vi "Test Boolean Event.vi"() -> ()   [LabVIEW 2021]
uses:
  Source/Omni-Bus/Omni_Bus.lvclass
  Source/Event Bus/Event_Bus.lvclass
  C:/TSA/Omni-Bus/Source/Omni-Bus/Bus Access/Bus_Access.lvclass
  Source/Local Bus/Local Bus.lvclass
  Source/Local Bus/Support/Tag List Type.ctl
  <vilib>/Utility/Data Type/Type Definitions/Data Type.ctl
  <vilib>/TSA/Abstract Data Classes/Abs_Types/Type/Abs_Type.lvclass/Abs_Type.ctl
  Source/Omni-Bus/Omni_Bus.lvclass/Omni_Bus.ctl
  Source/Omni-Bus/Support/Write/Write Boolean.vi
  Source/Omni-Bus/Support/Read/Read Boolean.vi
  Source/Omni-Bus/Support/FindVar.vi
  <vilib>/Utility/error.llb/Clear Errors.vi
  Source/Omni-Bus/Properties/Read Var Map.vi
  <vilib>/TSA/Abstract Data Classes/Abs_Types/Type/Properties/Read Tag.vi
  <vilib>/TSA/Abstract Data Classes/Abs_Types/Boolean/Abs_Boolean.lvclass
  C:/Program Files (x86)/National Instruments/LabVIEW 2021/vi.lib/TSA/Abstract Data Classes/Abs_Types/Type/Abs_Type.lvclass
  <vilib>/TSA/Abstract Data Classes/Abs_Types/Value/Abs_Value.lvclass
  Source/Omni-Bus/Support/Check For Read Only Error.vi
  Source/Omni-Bus/Support/Incorrect Tag String Error.vi
  <vilib>/TSA/Abstract Data Classes/Abs_Types/Type/Abs_Type.lvclass
  <vilib>/Utility/Data Type/NI_Data Type.lvlib
panel:
  in  "stop 6":bool
  out "Numeric 6":i32
  in  "Boolean 6":bool
  in  "stop 5":bool
  out "Numeric 5":i32
  out "Boolean 5":bool
  in  "stop 4":bool
  out "Numeric 4":i32
  out "Boolean 4":bool
  in  "stop 3":bool
  out "Numeric 3":i32
  out "Boolean 3":bool
  out "Boolean 2":bool
  in  "Boolean":bool
  out "Numeric 2":i32
  out "Numeric":i32
  in  "stop 2":bool
  in  "stop":bool
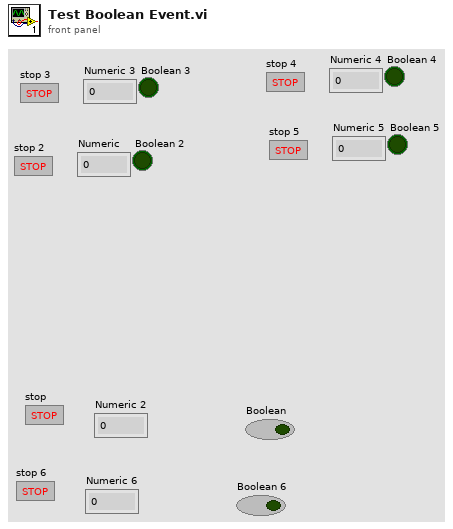
[diagram p1: front panel]
types:
  T1 = typedef "Local Bus.lvclass/Tag List Type.ctl" = cluster{"Tag":string, "Type":T2}
  T2 = typedef "NI_Data Type.lvlib/Data Type.ctl" = enum8{"Invalid Type", "Void", "I8", "I16", "I32", "I64", "U8", "U16", "U32", "U64", "Single Float", "Double Float", "Extended Float", "Single Complex", "Double Complex", "Extended Complex", "Enum U8", "Enum U16", "Enum U32", "Enum U64", "Single Float With Unit", "Double Float With Unit", "Extended Float With Unit", "Single Complex with Unit", "Double Complex with Unit", "Extended Complex with Unit", "Boolean", "String", "Path", "Picture", "Tag", "Array", "Cluster", "Variant", "LV Variant", "Waveform", "Timestamp", "Digital Waveform", "Digital Data", "ExpressData", "Refnum", "External Data", "VI", "Poly VI", "LabVIEW Class Instance", "Fixed Point", "Set Collection", "Map Collection"}
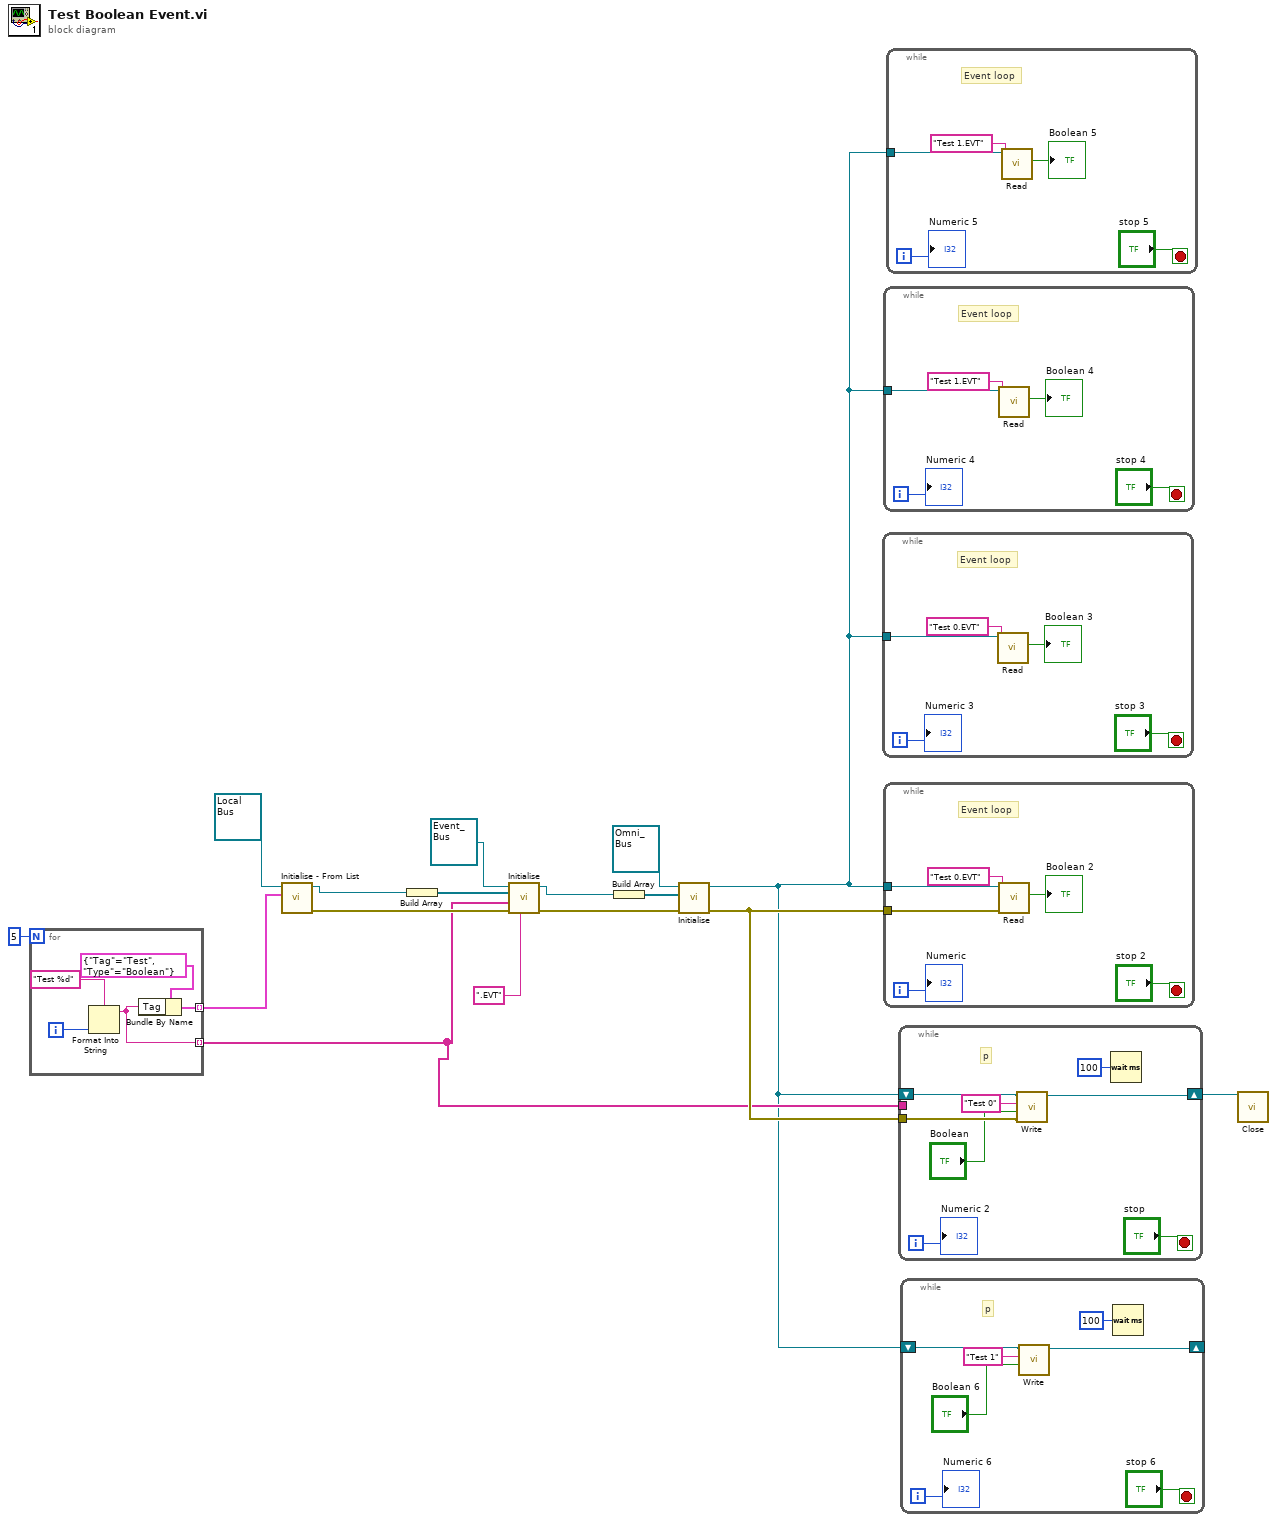
[diagram p0: block diagram]
diagram:
  n1 = for {
    N: 5 -> [_]
    tunnel: [w18] -> w4 mode=indexing
    tunnel: [w17] -> w3 mode=indexing
    i -> [w19]
    n2 = Format Into String(format string="Test %d", w19) -> (resulting string=w17:string)  [unwired: 2 in, 1 out]
    n3 = Bundle By Name(cluster=T1 {"Tag"="Test", "Type"=enum."Boolean"} ("Cluster"), "Tag"=w17) -> (w18:T1)
  }
  n4 = call "Initialise - From List.vi"("Tag List"=w4, "Local Bus in"=refnum<class "Local Bus.lvclass"> refnum) -> ("error out"=w9:errorcluster, "Local Bus out"=w8:refnum<class "Local Bus.lvclass">)  [unwired: 8 in]
  n5 = Build Array(w8) -> (w10:refnum<class "Local Bus.lvclass">[])
  n6 = call "Initialise.vi"("Tag Root"=".EVT", "error in (no error)"=w9, "Tags to Event"=w3, "Buses"=w10, "Event_Bus in"=refnum<class "Event_Bus.lvclass"> refnum) -> ("error out"=w13:errorcluster, "Event_Bus out"=w12:refnum<class "Event_Bus.lvclass">)  [unwired: 5 in]
  n7 = Build Array(w12) -> (w14:refnum<class "Event_Bus.lvclass">[])
  n8 = call-dynamic "Initialise.vi"("error in (no error)"=w13, "Bus Access"=w14, "Var Bus in"=refnum<class "Omni_Bus.lvclass"> refnum) -> ("error out"=w15:errorcluster, "Var Bus out"=w1:refnum<class "Omni_Bus.lvclass">)  [unwired: 7 in]
  n9 = while {
    tunnel: w1 -> [w26]
    i -> [w24]
    stop <- "stop 3" stop-if-true
    # "Event loop"
    n10 = call-poly "Read.vi"("Tag"="Test 0.EVT", "Var Bus in"=w26) -> ("Boolean"=→"Boolean 3":bool)  [unwired: 7 in, 2 out]
    "Numeric 3" <- w24
  }
  n11 = while {
    tunnel: w1 -> [w31]
    i -> [w29]
    stop <- "stop 4" stop-if-true
    # "Event loop"
    n12 = call-poly "Read.vi"("Tag"="Test 1.EVT", "Var Bus in"=w31) -> ("Boolean"=→"Boolean 4":bool)  [unwired: 7 in, 2 out]
    "Numeric 4" <- w29
  }
  n13 = while {
    tunnel: w1 -> [w37]
    tunnel: w15 -> [w36]
    i -> [w34]
    stop <- "stop 2" stop-if-true
    # "Event loop"
    n14 = call-poly "Read.vi"("error in (no error)"=w36, "Tag"="Test 0.EVT", "Var Bus in"=w37) -> ("Boolean"=→"Boolean 2":bool)  [unwired: 6 in, 2 out]
    "Numeric" <- w34
  }
  n15 = while {
    tunnel: w1 -> [w42]
    i -> [w40]
    stop <- "stop 5" stop-if-true
    # "Event loop"
    n16 = call-poly "Read.vi"("Tag"="Test 1.EVT", "Var Bus in"=w42) -> ("Boolean"=→"Boolean 5":bool)  [unwired: 7 in, 2 out]
    "Numeric 5" <- w40
  }
  n17 = while {
    tunnel: w15 -> [w48]
    shift-right: [w45] -> w6
    shift-left: w1 -> [w49]
    tunnel: w3 -> [_]
    i -> [w47]
    stop <- "stop" stop-if-true
    # "p"
    n18 = call-poly "Write.vi"("error in (no error)"=w48, "Boolean"="Boolean", "Tag"="Test 0", "Omni_Bus in"=w49) -> ("Omni_Bus out"=w45:refnum<class "Omni_Bus.lvclass">)  [unwired: 6 in, 1 out]
    n19 = Wait (ms)(milliseconds to wait=u32 100) -> ()  [unwired: 1 out]
    "Numeric 2" <- w47
  }
  n20 = while {
    shift-right: [w53] -> _
    shift-left: w1 -> [w56]
    i -> [w55]
    stop <- "stop 6" stop-if-true
    # "p"
    n21 = call-poly "Write.vi"("Boolean"="Boolean 6", "Tag"="Test 1", "Omni_Bus in"=w56) -> ("Omni_Bus out"=w53:refnum<class "Omni_Bus.lvclass">)  [unwired: 7 in, 1 out]
    n22 = Wait (ms)(milliseconds to wait=u32 100) -> ()  [unwired: 1 out]
    "Numeric 6" <- w55
  }
  n23 = call-dynamic "Close.vi"("Data in"=w6) -> ()  [unwired: 9 in, 2 out]
